vi "Calculate distance from sonar reading.vi"() -> (3 "Numeric":dbl)   [LabVIEW 2011]
uses:
  Robot Global Data.vi
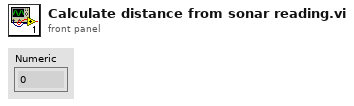
[diagram p1: front panel]
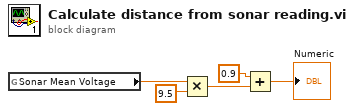
[diagram p0: block diagram]
diagram:
  n1 = global read "Robot Global Data.vi" "Sonar Mean Voltage"() -> (w2:dbl)
  n2 = Multiply(x=w2, y=9.5) -> (x*y=w3:dbl)
  n3 = Add(x=0.9, y=w3) -> (x+y=→"Numeric":dbl)
